vi "get_previous.vi"(8 "error in (no error)":errorcluster, 11 "Iterator in":refnum<class "Iterator.lvclass">) -> (0 "error out":errorcluster, 1 "found?":bool, 2 "previous":refnum<class "Iterator.lvclass">, 3 "Iterator out":refnum<class "Iterator.lvclass">)   [LabVIEW 2021, in "Iterator.lvclass"]
uses:
  Iterator.lvclass
  Iterator.lvclass/Iterator.ctl
  IDoublyNode/IDoublyNode.lvclass
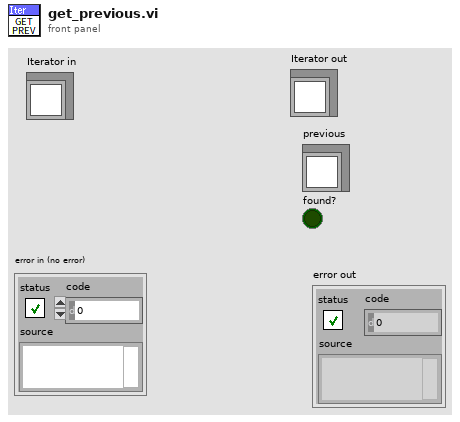
[diagram p1: front panel]
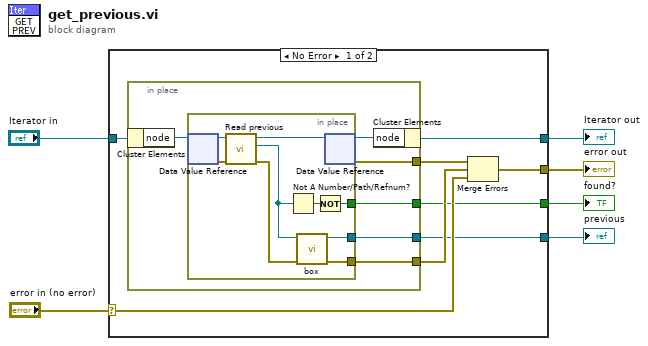
[diagram p0: block diagram]
diagram:
  n1 = case shown="No Error" "error in (no error)" {
    selector: "error in (no error)" -> [w13 w31]
    tunnel: [w12 w31] -> w5
    tunnel: "Iterator in" -> [w14 w30]
    tunnel: [w9 _] -> w2
    tunnel: [w8 _] -> w3
    tunnel: [w7 w30] -> w1
    frame No Error {
      n2 = in-place {
        in-place-border: [w18] -> w8
        in-place-border: [w17] -> w10
        in-place-border: [w16] -> w11
        in-place-border: [w15] -> w9
        n3 = in-place-cluster #1(w14) -> ("node"=w20:refnum<data-value>)
        n4 = in-place {
          in-place-border: [w29] -> w18
          in-place-border: [w28] -> w17
          in-place-border: [w26] -> w15
          n5 = in-place-dvr #2(w20) -> (w25:refnum<class "IDoublyNode.lvclass">, w24:errorcluster)
          n6 = call-dynamic "Read previous.vi"("error in (no error)"=w24, "NodeType in"=w25) -> ("error out"=w23:errorcluster, "previous"=w22:refnum<data-value>, "NodeType out"=w21:refnum<class "IDoublyNode.lvclass">)  [unwired: 7 in]
          n7 = Not A Number/Path/Refnum?(number/path/refnum=w22) -> (NaN/Path/Refnum?=w27:bool)
          n8 = call "box.vi"("error in (no error)"=w23, "node"=w22) -> ("error out"=w28:errorcluster, "Iterator out"=w29:refnum<class "Iterator.lvclass">)  [unwired: 8 in]
          n9 = Not(x=w27) -> (.not. x?=w26:bool)
          n10 = in-place-dvr #2(w21) -> (w19:refnum<data-value>, w16:errorcluster)
        }
        n11 = in-place-cluster #1("node"=w19) -> (w7:refnum<class "Iterator.lvclass">)
      }
      n12 = Merge Errors(w11, w10, w13) -> (w12:errorcluster)
    }
    frame Error {
    }
  }
  "error out" <- w5
  "previous" <- w3
  "found?" <- w2
  "Iterator out" <- w1
